vi "TestCOMXYZandrootXYZ2.vi"() -> ()   [LabVIEW 2012]
panel:
  out "自动化引用句柄":refnum<k7>
  in  "Z":dbl format="%#_13g"
  in  "Y":dbl format="%#_13g"
  in  "X":dbl format="%#_13g"
  out "XYZ":dbl
  out "CX":dbl
  in  "XYZandrootXYZ.IClass1":refnum<k7>
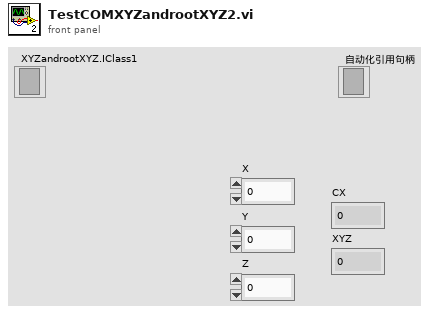
[diagram p1: front panel]
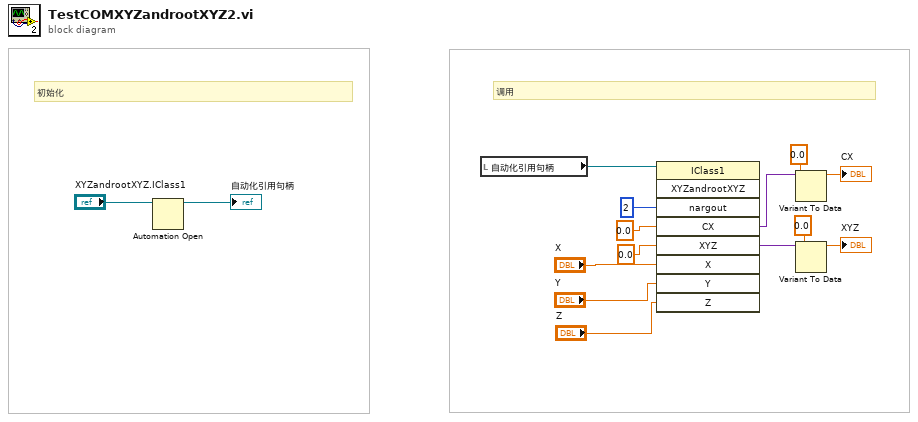
[diagram p0: block diagram]
diagram:
  # "调用"
  # "初始化"
  n1 = Automation Open(Automation Refnum="XYZandrootXYZ.IClass1") -> (Automation Refnum=→"自动化引用句柄":refnum<k7>)  [unwired: 3 in, 1 out]
  n2 = local read "自动化引用句柄"() -> (w1:refnum<k7>)
  n3 = invoke class="IClass1" method="XYZandrootXYZ"(reference=w1, "nargout"=2, "CX"=0.0, "XYZ"=0.0, "X"="X", "Y"="Y", "Z"="Z") -> ("CX"=w7:variant, "XYZ"=w6:variant)  [unwired: 2 in, 7 out]
  n4 = Variant To Data(type=0.0, Variant=w7) -> (data=→"CX":dbl)  [unwired: 1 in, 1 out]
  n5 = Variant To Data(type=0.0, Variant=w6) -> (data=→"XYZ":dbl)  [unwired: 1 in, 1 out]
